vi "getAllUserEventInstance.vi"(8 "error in (no error)":errorcluster, 11 "tcpServer in":refnum<class "TcpServer.lvclass">) -> (0 "error out":errorcluster, 2 "UserEvents":T1, 3 "tcpServer out":refnum<class "TcpServer.lvclass">)   [LabVIEW 2018, in "TcpServer.lvclass"]
doc: "Get all the user event instances."
uses:
  TcpServer.lvclass
  typedef/userEventsTypeDef.ctl
  typedef/packetConnIDTypeDef.ctl
  typedef/ackTypeDef.ctl
  typedef/eventConnIDTypeDef.ctl
  TcpServer.lvclass/TcpServer.ctl
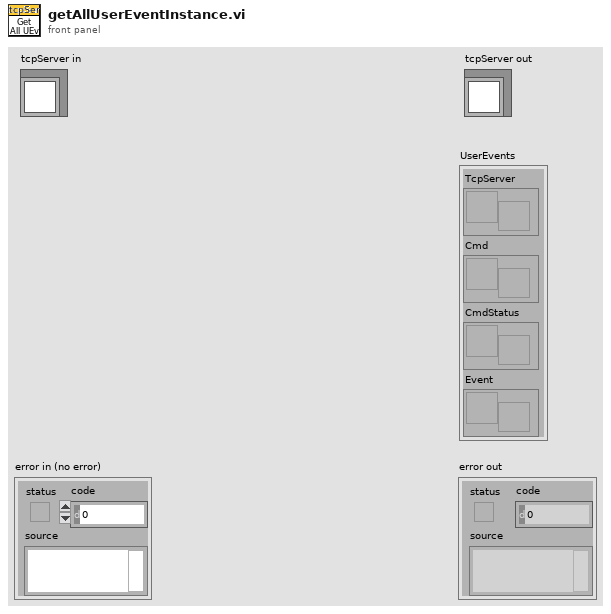
[diagram p1: front panel]
types:
  T1 = typedef "TcpServer.lvclass/userEventsTypeDef.ctl" = cluster{"TcpServer":refnum<user-event>, "Cmd":refnum<user-event>, "CmdStatus":refnum<user-event>, "Event":refnum<user-event>}
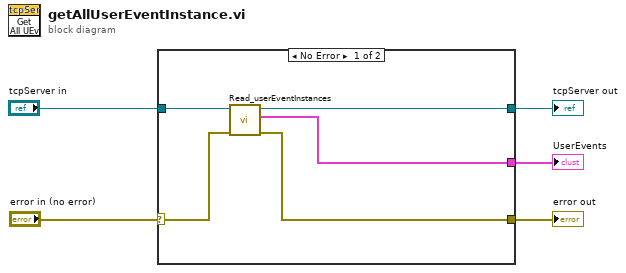
[diagram p0: block diagram]
diagram:
  n1 = case shown="No Error" "error in (no error)" {
    selector: "error in (no error)" -> [w8 w12]
    tunnel: [w7 w12] -> w4
    tunnel: [w9 w11] -> w2
    tunnel: "tcpServer in" -> [w10 w11]
    tunnel: [w6 _] -> w1
    frame No Error {
      n2 = call "Read_userEventInstances.vi"("error in (no error)"=w8, "tcpServer in"=w10) -> ("error out"=w7:errorcluster, "UserEvents"=w6:T1, "tcpServer out"=w9:refnum<class "TcpServer.lvclass">)  [unwired: 7 in]
    }
    frame Error {
    }
  }
  "error out" <- w4
  "tcpServer out" <- w2
  "UserEvents" <- w1
